vi "Goal-directed Line Following.vi"() -> ()   [LabVIEW 2018]
uses:
  <extravilib>/ChannelInstances/Tag-bool.lvlib
  <vilib>/Platform/TimedLoop/XDataNode/XDataNode.xnode
  <vilib>/Platform/TimedLoop/XDataNode/nitl_modes.ctl
  <vilib>/Platform/TimedLoop/XDataNode/XDNodeRunTimeDep.lvlib
  <vilib>/Platform/TimedLoop/XDataNode/wakeup.ctl
  <vilib>/Platform/TimedLoop/XDataNode/timing_clust.ctl
  <extravilib>/ChannelInstances/Tag-a[.](dbl).lvlib
  <extravilib>/ChannelInstances/Lossy Stream-a[.,.](dbl).lvlib
  <extravilib>/ChannelInstances/Tag-dbl.lvlib
  SubVIs/GDLF SM States.ctl
panel:
  in  "Hue Threshold":cluster{i32, i32}(slide)={0, 255} scale=0.0..255.0
  in  "Saturation Threshold":cluster{i32, i32}(slide)={0, 255} scale=0.0..255.0
  in  "Luminance Threshold":cluster{i32, i32}(slide)={0, 255} scale=0.0..255.0
  out "error out":errorcluster
  out "System State":T1
  out "Destination Task \nCoordinates (cm)":dbl[](array[numeric])
  in  "Stop Button":bool
  out "Calibrated":bool
  out "Information":string
  in  "GO?":bool
  out "Processed Image":T2(plugin-control)
  out "Desired Task \nCoordinates (cm)":dbl[](array[numeric])
  out "Current Task Coordinates (cm)":dbl[](array[numeric])
  out "Silk":T2(plugin-control)
  out "Original Acquired Image":T2(plugin-control)
  # "Mechatronic Systems Board"
  # "Goal-directed Line Following"
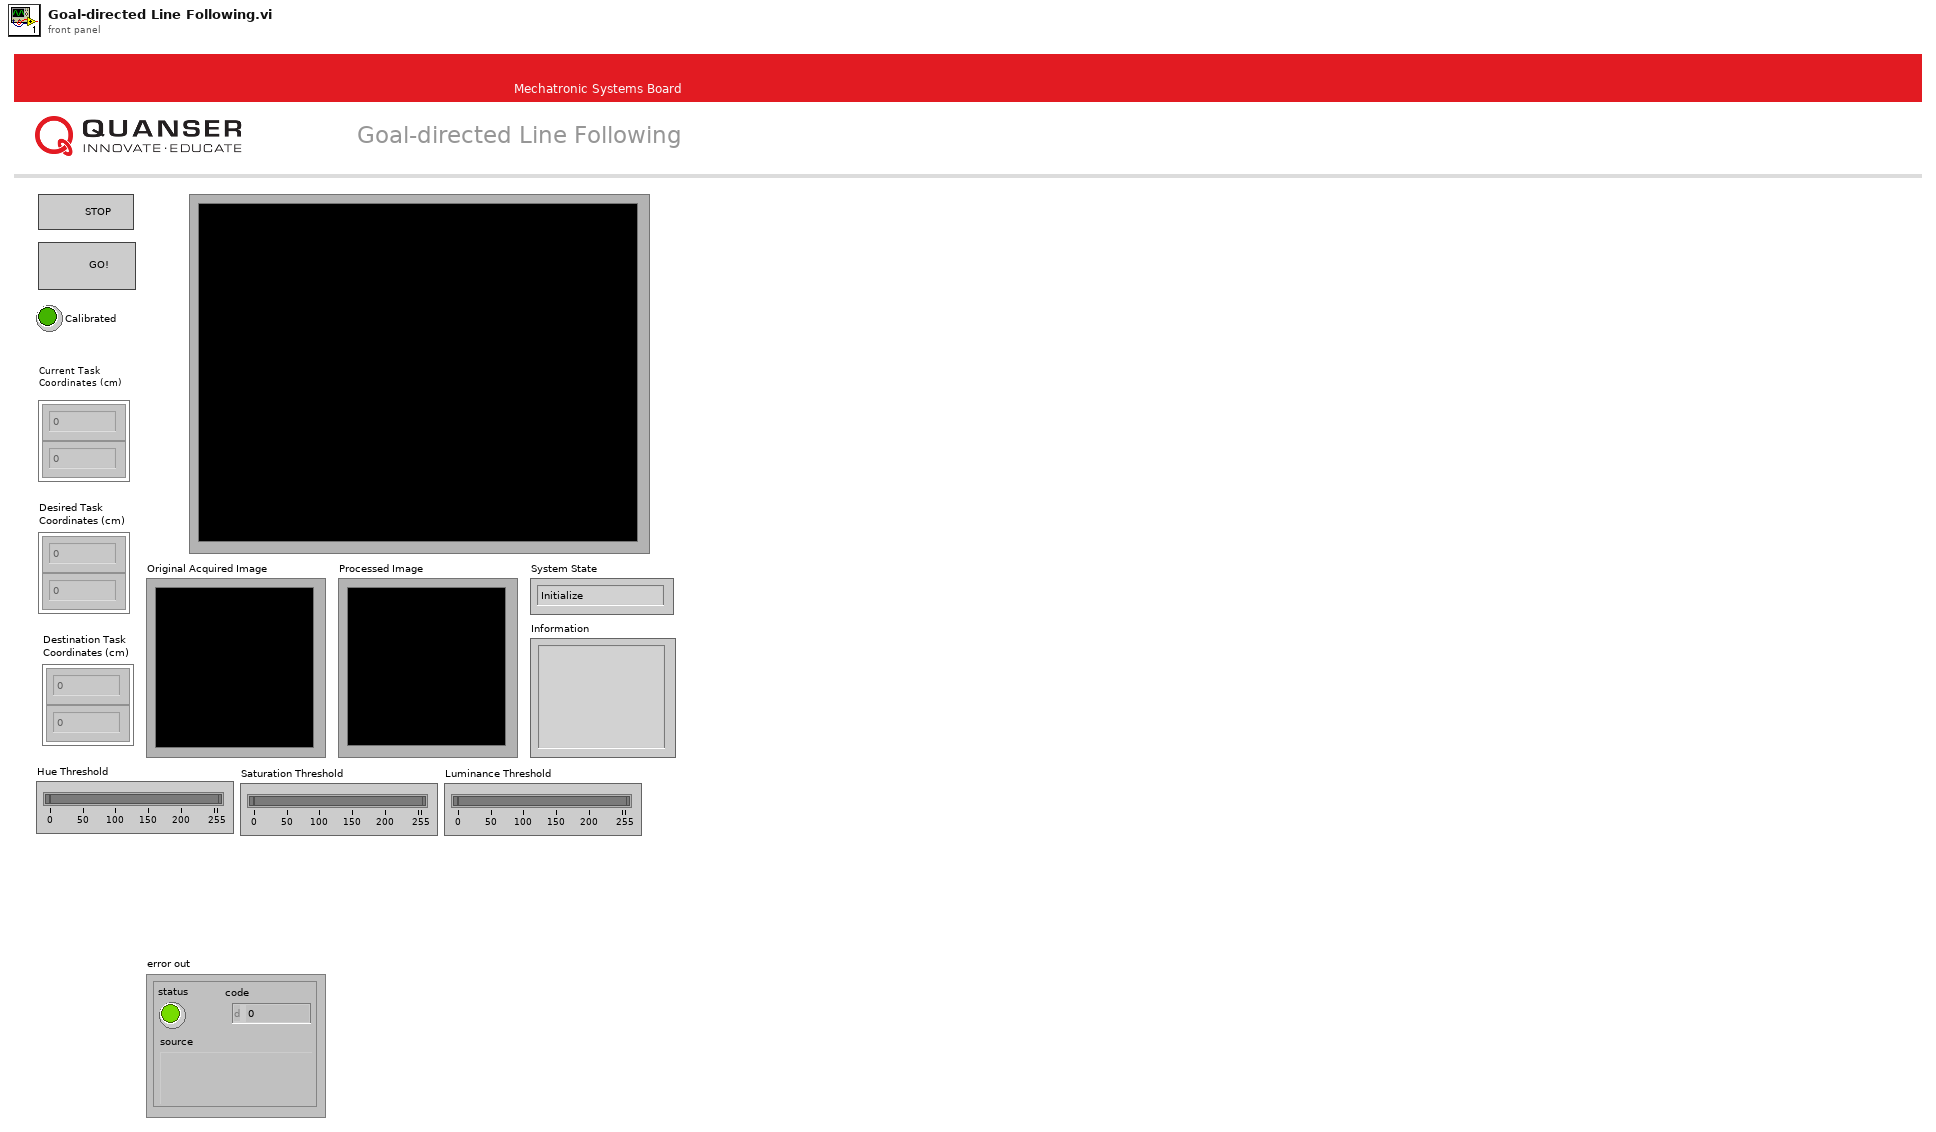
[diagram p1: front panel]
types:
  T1 = typedef "GDLF SM States.ctl" = enum16{"Initialize", "Set Destination", "Move", "Wait", "Backtrack", "Stop"}
  T2 = typedef "IMAQ Image.ctl" = refnum<image>
  T3 = typedef "QNET MS IO Cluster.ctl" = cluster{"Error":errorcluster, "Encoder Calibration Values":i32[], "Update Calibration":bool, "JPEG Resolutions":u16, "Raw Resolutions":u16, "Image Mode":enum16{"RAW RGB", "RAW Gray Scale", "JPEG"}, "FPGA Ref":refnum<k20>}
  T4 = typedef "XDNodeRunTimeDep.lvlib/timing_clust.ctl" = cluster{"Expected End [f-1]":u64, "Actual End [f-1]":u64, "Finished Late? [f-1]":bool, "Expected End [i-1]":u64, "Actual End [i-1]":u64, "Finished Late? [i-1]":bool, "Expected Start [i]":u64, "Actual Start [i]":u64, "Expected Start [f]":u64, "Actual Start [f]":u64, "Source Name":string, "Structure Name":string, "Period":i64, "Deadline":i64, "Offset":i64, "Start":i64, "Priority":i32, "Timeout":i32, "Mode":T5, "Wakeup Reason":T6, "Error":errorcluster, "Source Type":string, "Secondary Source Type":string, "Global End Time":u64, "Global Start Time":u64, "Frame Duration":u64, "Iteration Duration":u64, "Assigned CPU":i32, "I/O Scan Engine Mode":u32}
  T5 = typedef "XDNodeRunTimeDep.lvlib/nitl_modes.ctl" = enum32{"No Change", "Process missed periods, maintain original phase", "Discard missed periods, maintain original phase", "Process missed periods, ignore original phase", "Discard missed periods, ignore original phase"}
  T6 = typedef "XDNodeRunTimeDep.lvlib/wakeup.ctl" = enum32{"Normal", "Aborted", "Asynchronous wakeup", "Timing source error", "Timed loop error", "Timeout"}
  T7 = typedef "Tag-a[.](dbl).lvlib/))Channel.ctl" = refnum<queue>
  T8 = typedef "Tag-bool.lvlib/))Channel.ctl" = refnum<queue>
  T9 = typedef "ROI Descriptor" = cluster{"Global Rectangle":i32[], "Contours":cluster{"ID":enum32{"External", "Internal"}, "Type":u32, "Coordinates":i32[]}[]}
  T10 = cluster{"Hue Threshold":cluster{i32, i32}, "Saturation Threshold":cluster{i32, i32}, "Luminance Threshold":cluster{i32, i32}}
  T11 = typedef "Lossy Stream-a[.,.](dbl).lvlib/)Channel.ctl" = refnum<queue>
  T12 = cluster{"Global Rectangle":i32[], "Contours":cluster{"Contour Type":u32, "ROI Type":u32, "Points":i32[]}[]}
  T13 = typedef "Tag-dbl.lvlib/))Channel.ctl" = refnum<queue>
  T14 = cluster{"Contour Type":u32, "ROI Type":u32, "Points":i32[]}[]
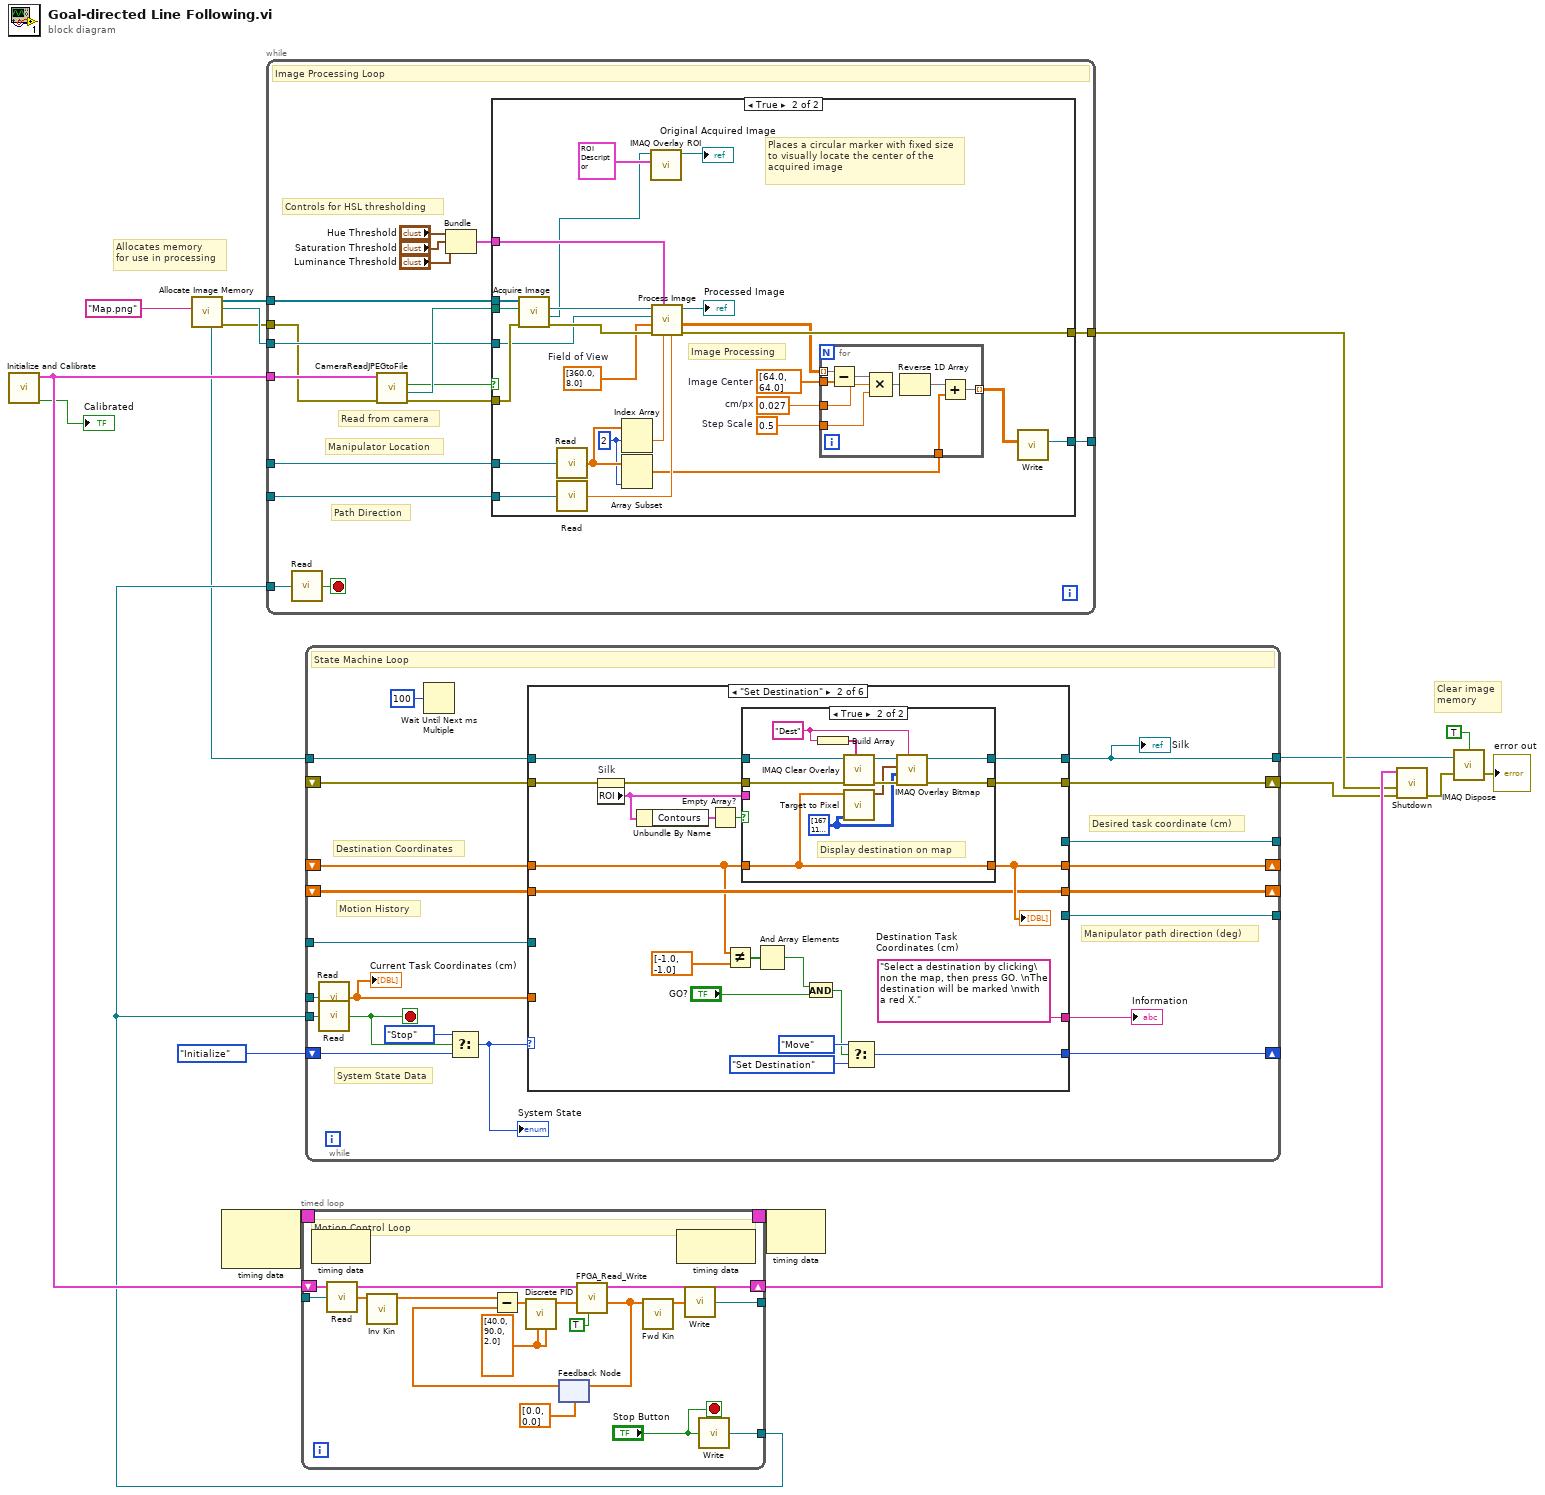
[diagram p0: block diagram]
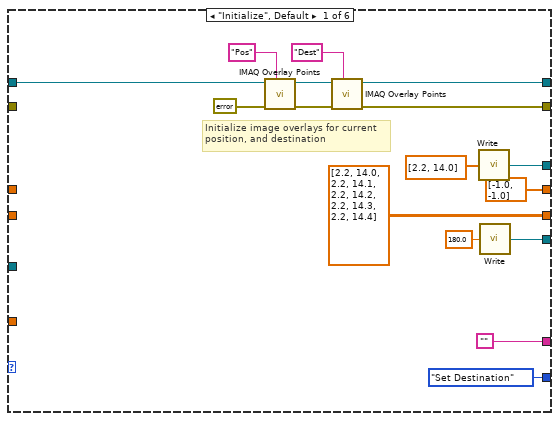
[diagram p2: hidden frame]
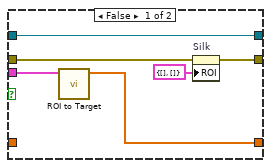
[diagram p3: hidden frame]
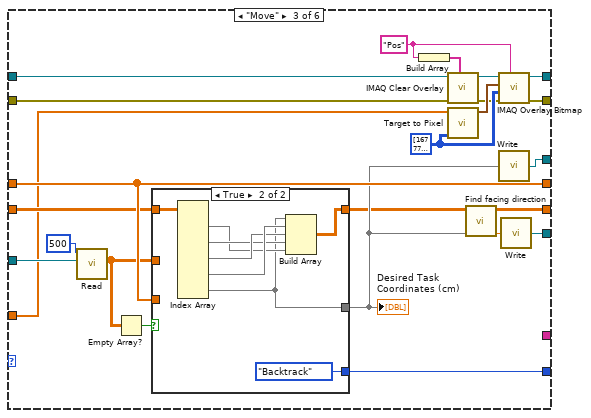
[diagram p4: hidden frame]
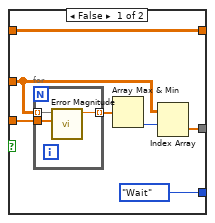
[diagram p5: hidden frame]
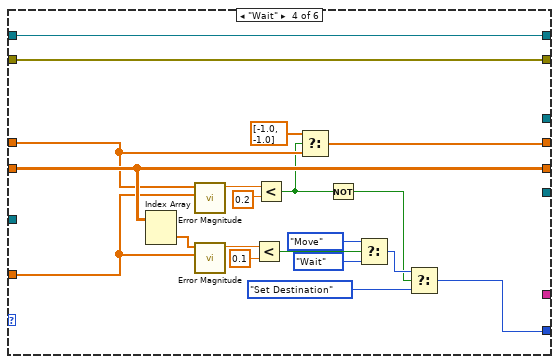
[diagram p6: hidden frame]
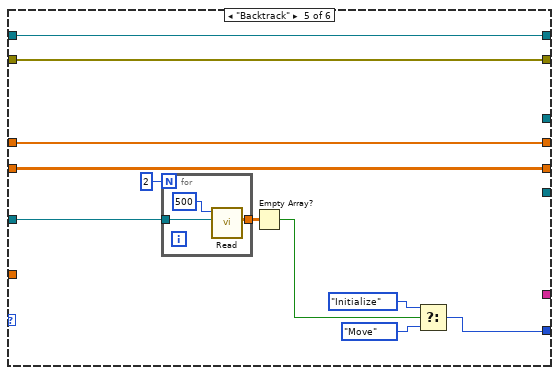
[diagram p7: hidden frame]
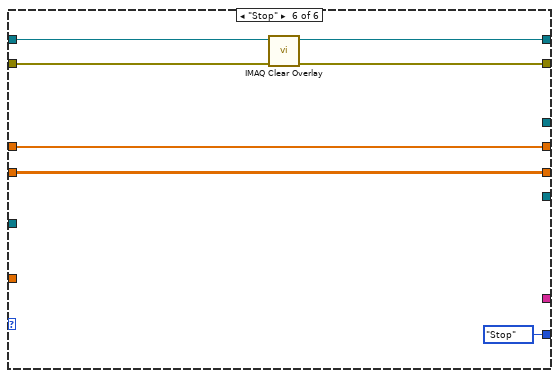
[diagram p8: hidden frame]
diagram:
  # "Allocates memory\nfor use in processing"
  # "Clear image\nmemory"
  n1 = call "Initialize and Calibrate.vi"() -> ("Calibrated"=→"Calibrated":bool, "IO Cluster"=w11:T3)  [unwired: 10 in]
  n2 = call "Allocate Image Memory.vi"("Base Image File"="Map.png") -> ("error out"=w15:errorcluster, "HSL Threshold"=w16:T2, "Acquisition Memory"=w17:T2[], "Base Image"=w2:T2)  [unwired: 5 in, 2 out]
  n3 = node-c288() -> (w14:T4)  [unwired: 2 in]
  n4 = timed-loop {
    timing: w14 -> [_]
    timing-out: [_] -> w13
    tunnel: [w25] -> _
    tunnel: _ -> [w24]
    shift-right: [w30] -> w12
    shift-left: w11 -> [w22]
    tunnel: [w20] -> w4
    stop <- "Stop Button" stop-if-true
    w19 = dbl[] [40.0, 90.0, 2.0] ("Gains Motor 0")
    # "Motion Control Loop"
    n5 = node-c288() -> ()  [unwired: 1 in, 1 out]
    n6 = call <extravilib>:"Read.vi"("channel"=w24) -> ("element"=w23:dbl[])  [unwired: 1 in, 1 out]
    n7 = call "Inv Kin.vi"("Task Coordinates (cm)"=w23) -> ("Joint Coordinates (rad)"=w31:dbl[])  [unwired: 10 in]
    n8 = feedback #1(dbl[] [0.0, 0.0] ("Joint Coordinates (rad)")) -> (w29:dbl[])
    n9 = Subtract(x=w31, y=w29) -> (x-y=w32:dbl[])
    n10 = call "Discrete PID.vi"("Gains Motor 1"=w19, "Gains Motor 0"=w19, "Error Array"=w32) -> ("Voltage"=w33:dbl[])  [unwired: 8 in]
    n11 = call "FPGA_Read_Write.vi"("Motors enabled?"=TRUE, "Commands"=w33, "IO Cluster In"=w22) -> ("Joint Coordinates (rad)"=w28:dbl[], "IO Cluster Out"=w30:T3)  [unwired: 5 in, 2 out]
    n12 = feedback-in #1(w28) -> ()
    n13 = call "Fwd Kin.vi"("Joint Coordinates (rad)"=w28) -> ("Task Coordinates (cm)"=w26:dbl[])  [unwired: 9 in, 1 out]
    n14 = node-c288() -> ()  [unwired: 1 in, 1 out]
    n15 = call <extravilib>:"Write.vi"("element"=w26) -> ("channel"=w25:T7)  [unwired: 1 out]
    n16 = call <extravilib>:"Write.vi"("element"="Stop Button") -> ("channel"=w20:T8)  [unwired: 1 out]
  }
  n17 = while {
    tunnel: w11 -> [w53]
    tunnel: [w49] -> w8
    tunnel: w17 -> [w48]
    tunnel: w16 -> [w47]
    tunnel: w15 -> [w46]
    tunnel: [w45] -> _
    tunnel: _ -> [w43]
    tunnel: _ -> [w44]
    tunnel: w4 -> [w42]
    stop <- w41 stop-if-true
    # "Path Direction"
    # "Controls for HSL thresholding"
    # "Read from camera"
    # "Manipulator Location"
    # "Image Processing Loop"
    n18 = call <extravilib>:"Read.vi"("channel"=w42) -> ("element"=w41:bool)  [unwired: 1 in, 1 out]
    n19 = call "CameraReadJPEGtoFile.vi"("error in"=w46, "IO Cluster In"=w53) -> ("Error Out"=w50:errorcluster, "Image File"=w52:path, "New Image Data"=w51:bool)  [unwired: 6 in, 1 out]
    n20 = Bundle("Hue Threshold"="Hue Threshold", "Saturation Threshold"="Saturation Threshold", "Luminance Threshold"="Luminance Threshold") -> (w37:T10)  [unwired: 1 in]
    n21 = case shown="True" w51 {
      tunnel: w52 -> [_ w78]
      tunnel: w50 -> [w54 w79]
      tunnel: [w54 w74] -> w49
      tunnel: w48 -> [_ w77]
      tunnel: w47 -> [_ w69]
      tunnel: [_ w66] -> w45
      tunnel: w44 -> [_ w60]
      tunnel: w43 -> [_ w59]
      tunnel: w37 -> [_ w58]
      frame False {
      }
      frame True {
        w64 = 2 ("index")
        w67 = 0.5  # Step Scale
        w72 = 0.027  # cm/px
        w71 = dbl[] [64.0, 64.0]  # Image Center
        w73 = dbl[] [360.0, 8.0]  # Field of View
        # "Image Processing"
        # "Places a circular marker with fixed size to visually locate the center of the acquired image"
        n22 = call "Acquire Image.vi"("Error In"=w79, "File Path"=w78, "Acquisition Memory"=w77) -> ("Error Out"=w75:errorcluster, "Source Image"=w55:T2, "HSL Image"=w56:T2)  [unwired: 4 in, 2 out]
        n23 = call <extravilib>:"Read.vi"("channel"=w59) -> ("element"=w65:dbl[])  [unwired: 1 in, 1 out]
        n24 = call <extravilib>:"Read.vi"("channel"=w60) -> ("element"=w63:dbl)  [unwired: 1 in, 1 out]
        n25 = Index Array(array=w65, index #1=w64) -> (element #1=w62:dbl)  [unwired: 1 in, 1 out]
        n26 = Array Subset(array=w65, length=w64) -> (w61:dbl[])  [unwired: 1 in]
        n27 = call "IMAQ Overlay ROI"("ROI Descriptor"=T9 {"Global Rectangle"=[16, 0, 145, 129], "Contours"=[{"ID"=enum."External", "Type"=7, "Coordinates"=[64, 64, 7, 8, 0, 0]}]}, "Image"=w55) -> ("Image Out"=→"Original Acquired Image":T2)  [unwired: 8 in, 1 out]
        n28 = call "Process Image.vi"("Path Angle"=w63, "Camera Angle"=w62, 7:w58, "Error In"=w75, "FOV"=w73, "Process Memory"=w69, "Acquired Image"=w56) -> ("Error Out"=w74:errorcluster, "Particle Locations"=w70:dbl[][], "Processed Image"=→"Processed Image":T2)  [unwired: 2 in]
        n29 = for {
          tunnel: w71 -> [w89]
          tunnel: [w87] -> w68 mode=indexing
          tunnel: w70 -> [w86] mode=indexing
          tunnel: w72 -> [w85]
          tunnel: w61 -> [w82]
          tunnel: w67 -> [w81]
          n30 = Subtract(x=w86, y=w89) -> (x-y=w88:dbl[])
          n31 = Compound Arithmetic op=MULTIPLY(w88, w85, w81) -> (w84:dbl[])
          n32 = Reverse 1D Array(array=w84) -> (reversed array=w83:dbl[])
          n33 = Add(x=w83, y=w82) -> (x+y=w87:dbl[])
        }
        n34 = call <extravilib>:"Write.vi"("element"=w68) -> ("channel"=w66:T11)  [unwired: 8 in, 2 out]
      }
    }
  }
  n35 = while {
    tunnel: w4 -> [w110]
    shift-right: [w108] -> _
    shift-left: _ -> [w109]
    tunnel: _ -> [w105]
    tunnel: [w101] -> _
    tunnel: _ -> [w107]
    tunnel: [w102] -> _
    tunnel: w2 -> [w100]
    shift-right: [w104] -> _
    shift-left: _ -> [w103]
    shift-right: [w99] -> _
    shift-left: GDLF_SM_States."Initialize" ("System State") -> [w97]
    shift-right: [w93] -> w9
    shift-left: _ -> [w92]
    tunnel: [w90] -> w6
    stop <- w94 stop-if-true
    # "Manipulator path direction (deg)"
    # "Destination Coordinates"
    # "Motion History"
    # "Desired task coordinate (cm)"
    # "System State Data"
    # "State Machine Loop"
    n36 = call <extravilib>:"Read.vi"("channel"=w107) -> ("element"=w106:dbl[])  [unwired: 1 in, 1 out]
    "Current Task Coordinates (cm)" <- w106
    n37 = call <extravilib>:"Read.vi"("channel"=w110) -> ("element"=w94:bool)  [unwired: 1 in, 1 out]
    n38 = Wait Until Next ms Multiple(millisecond multiple=u32 100) -> ()  [unwired: 1 out]
    n39 = Select(t=GDLF_SM_States."Stop", s=w94, f=w97) -> (s? t:f=w96:T1)
    "System State" <- w96
    n40 = case shown="\"Set Destination\"" w96 {
      tunnel: w109 -> [_ w141 w169 w222 w233 w245]
      tunnel: [dbl[][] [[2.2, 14.0], [2.2, 14.1], [2.2, 14.2], [2.2, 14.3], [2.2, 14.4]] w141 w173 w222 w233 w245] -> w108
      tunnel: w106 -> [_ _ w164 w211 _ _]
      tunnel: w103 -> [_ w133 w180 w214 w235 w244]
      tunnel: w105 -> [_ _ w187 _ w231 _]
      tunnel: [dbl[] [-1.0, -1.0] ("Joint Coordinates (rad)") w146 w180 w213 w235 w244] -> w104
      tunnel: [w123 _ w186 _ _ _] -> w102
      tunnel: [w120 _ w185 _ _ _] -> w101
      tunnel: w100 -> [w118 w140 w184 w215 w234 w243]
      tunnel: [GDLF_SM_States."Set Destination" ("System State") w145 w167 w206 w226 GDLF_SM_States."Stop" ("System State")] -> w99
      tunnel: ["" "Select a destination by clicking\non the map, then press GO. \nThe destination will be marked \nwith a red X." _ _ _ _] -> w98
      tunnel: [w113 w138 w181 w216 w236 w240] -> w93
      tunnel: w92 -> [_ w142 w183 w216 w236 w242]
      tunnel: [w115 w137 w182 w215 w234 w241] -> w90
      frame "Initialize", Default {
        # "Initialize image overlays for current\nposition, and destination"
        n41 = call "IMAQ Overlay Points"("Group"="Pos", "error in (no error)"=errorcluster {"status"=FALSE, "code"=0, "source"=""} ("error out"), "Image"=w118) -> ("error out"=w114:errorcluster, "Image Out"=w116:T2)  [unwired: 7 in]
        n42 = call "IMAQ Overlay Points"("Group"="Dest", "error in (no error)"=w114, "Image"=w116) -> ("error out"=w113:errorcluster, "Image Out"=w115:T2)  [unwired: 7 in]
        n43 = call <extravilib>:"Write.vi"("element"=dbl[] [2.2, 14.0] ("Joint Coordinates (rad)")) -> ("channel"=w120:T7)  [unwired: 1 out]
        n44 = call <extravilib>:"Write.vi"("element"=180.0) -> ("channel"=w123:T13)  [unwired: 1 out]
      }
      frame "Set Destination" {
        n45 = property on="Silk" class="ImageControl"(error in=w142) -> (error out=w139:errorcluster, "ROI"=w134:T12)  [unwired: 1 in, 1 out]
        n46 = Unbundle By Name(w134) -> ("Contours"=w135:T14)
        n47 = Empty Array?(array=w135) -> (empty?=w136:bool)
        n48 = Not Equal?(x=w133, y=dbl[] [-1.0, -1.0] ("Joint Coordinates (rad)")) -> (x != y?=w129:bool[])
        n49 = case shown="True" w136 {
          tunnel: [w147 w159] -> w146
          tunnel: w140 -> [w149 w161]
          tunnel: w139 -> [w148 w156]
          tunnel: [w151 w155] -> w138
          tunnel: [w149 w160] -> w137
          tunnel: w133 -> [_ w159]
          tunnel: w134 -> [w152 _]
          frame False {
            n50 = call "ROI to Target.vi"("ROI"=w152) -> ("Target Coordinates"=w147:dbl[])  [unwired: 8 in, 2 out]
            n51 = property on="Silk" class="ImageControl"(error in=w148, "ROI"=T12 {"Global Rectangle"=[], "Contours"=[]}) -> (error out=w151:errorcluster)  [unwired: 1 in, 1 out]
          }
          frame True {
            w154 = "Dest" ("Group")
            w157 = u32[][] [[16711680, 16711680, 16777216, 16777216, 16777216, 16777216, 16777216, 16711680, 16711680], [16711680, 16711680, 16711680, 16777216, 16777216, 16777216, 16711680, 16711680, 16711680], [16777216, 16711680, 16711680, 16711680, 16777216, 16711680, 16711680, 16711680, 16777216], [16777216, 16777216, 16711680, 16711680, 16711680, 16711680, 16711680, 16777216, 16777216], [16777216, 16777216, 16777216, 16711680, 16711680, 16711680, 16777216, 16777216, 16777216], [16777216, 16777216, 16711680, 16711680, 16711680, 16711680, 16711680, 16777216, 16777216], [16777216, 16711680, 16711680, 16711680, 16777216, 16711680, 16711680, 16711680, 16777216], [16711680, 16711680, 16711680, 16777216, 16777216, 16777216, 16711680, 16711680, 16711680], [16711680, 16711680, 16777216, 16777216, 16777216, 16777216, 16777216, 16711680, 16711680]] ("Bitmap")
            # "Display destination on map"
            n52 = Build Array(w154) -> (w153:string[])
            n53 = call "IMAQ Clear Overlay"("Groups"=w153, "error in (no error)"=w156, "Image"=w161) -> ("error out"=w162:errorcluster, "Image Out"=w163:T2)  [unwired: 7 in]
            n54 = call "Target to Pixel.vi"("Symbol"=w157, "Target Coordinates"=w159) -> ("Target Pixel"=w158:cluster{"X":i32, "Y":i32})  [unwired: 9 in]
            n55 = call "IMAQ Overlay Bitmap"("Group"=w154, "error in (no error)"=w162, "Bitmap"=w157, "Top Left Point"=w158, "Image"=w163) -> ("error out"=w155:errorcluster, "Image Out"=w160:T2)  [unwired: 5 in]
          }
        }
        "Destination Task \nCoordinates (cm)" <- w146
        n56 = And Array Elements(Boolean array=w129) -> (logical AND=w128:bool)
        n57 = And(x=w128, y="GO?") -> (x .and. y?=w130:bool)
        n58 = Select(t=GDLF_SM_States."Move" ("System State"), s=w130, f=GDLF_SM_States."Set Destination" ("System State")) -> (s? t:f=w145:T1)
      }
      frame "Move" {
        w175 = "Pos" ("Group")
        w178 = u32[][] [[16777216, 16777216, 6618880, 16777216, 6618880, 16777216, 6618880, 16777216, 16777216], [16777216, 6618880, 16777216, 6618880, 16777216, 6618880, 16777216, 6618880, 16777216], [6618880, 16777216, 6618880, 16777216, 6618880, 16777216, 6618880, 16777216, 6618880], [16777216, 6618880, 16777216, 6618880, 16777216, 6618880, 16777216, 6618880, 16777216], [6618880, 16777216, 6618880, 16777216, 6618880, 16777216, 6618880, 16777216, 6618880], [16777216, 6618880, 16777216, 6618880, 16777216, 6618880, 16777216, 6618880, 16777216], [6618880, 16777216, 6618880, 16777216, 6618880, 16777216, 6618880, 16777216, 6618880], [16777216, 6618880, 16777216, 6618880, 16777216, 6618880, 16777216, 6618880, 16777216], [16777216, 16777216, 6618880, 16777216, 6618880, 16777216, 6618880, 16777216, 16777216]] ("Bitmap")
        n59 = call <extravilib>:"Read.vi"("channel"=w187, "timeout in ms (-1)"=500) -> ("element"=w170:dbl[][])  [unwired: 4 in, 5 out]
        n60 = Empty Array?(array=w170) -> (empty?=w165:bool)
        n61 = case shown="True" w165 {
          tunnel: w170 -> [w192 _]
          tunnel: w180 -> [w191 _]
          tunnel: [w190 w199] -> w171
          tunnel: w169 -> [w189 w204]
          tunnel: [w189 w198] -> w168
          tunnel: [GDLF_SM_States."Wait" ("System State") GDLF_SM_States."Backtrack" ("System State")] -> w167
          frame False {
            n62 = for {
              tunnel: w192 -> [w197] mode=indexing
              tunnel: [w196] -> w194 mode=indexing
              tunnel: w191 -> [w195]
              n63 = call "Error Magnitude.vi"("Actual Task Coordinates (cm)"=w195, "Desired Task Coordinates (cm)"=w197) -> ("Task-space\nError"=w196:dbl)  [unwired: 9 in]
            }
            n64 = Array Max & Min(array=w194) -> (min index (indices)=w193:i32)  [unwired: 3 out]
            n65 = Index Array(array=w192, index (row)=w193) -> (element=w190:dbl[])  [unwired: 1 in]
          }
          frame True {
            n66 = Index Array(array=w204) -> (element #1=w200:dbl[], element #2=w201:dbl[], element #3=w202:dbl[], element #4=w203:dbl[], element #5=w199:dbl[])  [unwired: 10 in]
            n67 = Build Array(w199, w203, w202, w201, w200) -> (w198:dbl[][])
          }
        }
        "Desired Task \nCoordinates (cm)" <- w171
        n68 = Build Array(w175) -> (w174:string[])
        n69 = call "IMAQ Clear Overlay"("Groups"=w174, "error in (no error)"=w183, "Image"=w184) -> ("error out"=w176:errorcluster, "Image Out"=w177:T2)  [unwired: 7 in]
        n70 = call "Target to Pixel.vi"("Symbol"=w178, "Target Coordinates"=w164) -> ("Target Pixel"=w179:cluster{"X":i32, "Y":i32})  [unwired: 9 in]
        n71 = call "Find facing direction.vi"("Desired Task Coordinates (cm)"=w171, "Motion History In"=w168) -> ("Facing Direction (deg)"=w172:dbl, "Motion History Out"=w173:dbl[][])  [unwired: 8 in]
        n72 = call "IMAQ Overlay Bitmap"("Group"=w175, "error in (no error)"=w176, "Bitmap"=w178, "Top Left Point"=w179, "Image"=w177) -> ("error out"=w181:errorcluster, "Image Out"=w182:T2)  [unwired: 5 in]
        n73 = call <extravilib>:"Write.vi"("element"=w171) -> ("channel"=w185:T7)  [unwired: 1 out]
        n74 = call <extravilib>:"Write.vi"("element"=w172) -> ("channel"=w186:T13)  [unwired: 1 out]
      }
      frame "Wait" {
        n75 = Index Array(array=w222) -> (element=w225:dbl[])  [unwired: 2 in]
        n76 = call "Error Magnitude.vi"("Actual Task Coordinates (cm)"=w211, "Desired Task Coordinates (cm)"=w214) -> ("Task-space\nError"=w218:dbl)  [unwired: 9 in]
        n77 = call "Error Magnitude.vi"("Actual Task Coordinates (cm)"=w211, "Desired Task Coordinates (cm)"=w225) -> ("Task-space\nError"=w224:dbl)  [unwired: 9 in]
        n78 = Less?(x=w224, y=0.1) -> (x < y?=w220:bool)
        n79 = Less?(x=w218, y=0.2) -> (x < y?=w208:bool)
        n80 = Select(t=dbl[] [-1.0, -1.0], s=w208, f=w214) -> (s? t:f=w213:dbl[])
        n81 = Not(x=w208) -> (.not. x?=w207:bool)
        n82 = Select(t=GDLF_SM_States."Move", s=w220, f=GDLF_SM_States."Wait") -> (s? t:f=w210:T1)
        n83 = Select(t=w210, s=w207, f=GDLF_SM_States."Set Destination" ("t")) -> (s? t:f=w206:T1)
      }
      frame "Backtrack" {
        n84 = for {
          N: 2 -> [_]
          tunnel: w231 -> [w239]
          tunnel: [w238] -> w230
          n85 = call <extravilib>:"Read.vi"("channel"=w239, "timeout in ms (-1)"=500) -> ("element"=w238:dbl[][])  [unwired: 4 in, 5 out]
        }
        n86 = Empty Array?(array=w230) -> (empty?=w229:bool)
        n87 = Select(t=GDLF_SM_States."Initialize" ("System State"), s=w229, f=GDLF_SM_States."Move") -> (s? t:f=w226:T1)
      }
      frame "Stop" {
        n88 = call "IMAQ Clear Overlay"("error in (no error)"=w242, "Image"=w243) -> ("error out"=w240:errorcluster, "Image Out"=w241:T2)  [unwired: 8 in]
      }
    }
    "Information" <- w98
    "Silk" <- w90
  }
  n89 = node-c288(w13) -> ()  [unwired: 1 out]
  n90 = call "Shutdown.vi"("Image Processing Loop"=w9, "Manipulator Loop"=w8, "IO Cluster In"=w12) -> ("Error"=w7:errorcluster)  [unwired: 8 in]
  n91 = call "IMAQ Dispose"("All Images? (No)"=TRUE, "Image"=w6, "error in (no error)"=w7) -> ("error out"=→"error out":errorcluster)  [unwired: 3 in]
